vi "Lidar 관심범위 내 데이터(속도결정에 사용).vi"(3 "filter angle(plus)":dbl, 5 "Lidar 오브젝트화 후 배열":dbl[][](array[numeric])) -> (0 "theta":dbl[](array[numeric]), 1 "r":dbl[](array[numeric]), 2 "차량 진행 영역의 장애물":dbl[][](array[numeric]))   [LabVIEW 2016]
uses:
  <vilib>/imath/engines/lvmath2/RunTimeEngine/Managers/WorkSpace/UID Generator.vi
  <vilib>/imath/engines/lvmath2/RunTimeEngine/BuiltInFunctions/size/NIMS_I32Row=size(GM).vi
  <instcachedir>/0/NIMS_I32Row=size(GM)_10ACDCB9F1F84A7E9F42C91D87611FB5.lvgen/NIMS_I32Row=size(GM)_10ACDCB9F1F84A7E9F42C91D87611FB5_001.vi
  <vilib>/imath/engines/lvmath2/RunTimeEngine/RunTimeType/NIMS_RunTimeType_From StrictType (excl LVString).vi
  <instcachedir>/0/NIMS_RunTimeType_From StrictType (excl LVString)_BBF44FB49F834B71AF7A14CCEDF8BECD.lvgen/NIMS_RunTimeType_From StrictType (excl LVString)_BBF44FB49F834B71AF7A14CCEDF8BECD_000.vi
  <vilib>/imath/engines/lvmath2/RunTimeEngine/LocalVariableDefStatement/MC_LocalVariableDefStatement_Display.vi
  <vilib>/imath/engines/lvmath2/RunTimeEngine/IndexRead/NIMS M(S,S).vi
  <instcachedir>/0/NIMS M(S,S)_AC51E74150A542F7991B9634C66F3096.lvgen/NIMS M(S,S)_AC51E74150A542F7991B9634C66F3096_002.vi
  <vilib>/imathl/engines/lvmath/Functions/Error Handling/Create Error.vi
  <vilib>/imath/engines/lvmath2/RunTimeEngine/Managers/SymbolTable/Clear UID.vi
  <vilib>/imath/engines/lvmath2/RunTimeEngine/NodeEndStatement/NIMS_NodeEndStatement_Output.vi
  <instcachedir>/0/NIMS_NodeEndStatement_Output_53EC0D466D134D7ABD903AC30B43404B.lvgen/NIMS_NodeEndStatement_Output_53EC0D466D134D7ABD903AC30B43404B_010.vi
  <vilib>/imath/engines/lvmath2/RunTimeEngine/ErrorHandling/NIMS_Finalize Error.vi
  <vilib>/imath/engines/lvmath2/RunTimeEngine/IndexRead/NIMS M($,S).vi
  <instcachedir>/0/NIMS M($,S)_3E5749BBB62E49528D4765A77F1F6D98.lvgen/NIMS M($,S)_3E5749BBB62E49528D4765A77F1F6D98_000.vi
  <instcachedir>/0/NIMS_NodeEndStatement_Output_53EC0D466D134D7ABD903AC30B43404B.lvgen/NIMS_NodeEndStatement_Output_53EC0D466D134D7ABD903AC30B43404B_005.vi
  <vilib>/imath/engines/lvmath2/RunTimeEngine/Managers/SymbolTable/NIMS_WorkSpace.lvlib
panel:
  out "차량 진행 영역의 장애물 개수":i32
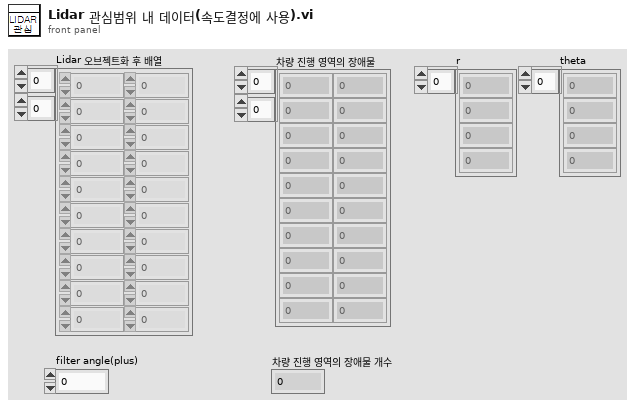
[diagram p1: front panel]
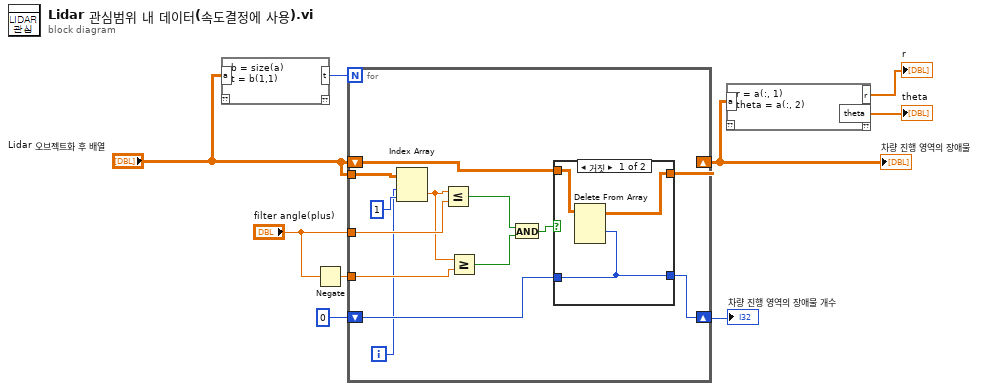
[diagram p0: block diagram]
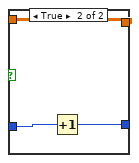
[diagram p2: hidden frame]
diagram:
  n1 = mathscript code="b = size(a)\nt = b(1,1)"("a"="Lidar 오브젝트화 후 배열") -> ("t"=w5:i32)  [unwired: 1 in, 1 out]
  n2 = Negate(x="filter angle(plus)") -> (-x=w8:dbl)
  n3 = for {
    N: w5 -> [_]
    tunnel: "filter angle(plus)" -> [w21]
    tunnel: w8 -> [w19]
    shift-right: [w12] -> w6
    shift-left: 0 ("비활성화된 인덱스 (행)") -> [w14]
    shift-right: [w13] -> w3
    shift-left: "Lidar 오브젝트화 후 배열" -> [w15]
    tunnel: "Lidar 오브젝트화 후 배열" -> [w11]
    i -> [w10]
    n4 = Index Array(array=w11, index (row)=w10, index (col)=1 ("비활성화된 인덱스 (열)")) -> (element=w20:dbl)
    n5 = Less Or Equal?(x=w20, y=w21) -> (x <= y?=w18:bool)
    n6 = Greater Or Equal?(x=w20, y=w19) -> (x >= y?=w17:bool)
    n7 = And(x=w18, y=w17) -> (x .and. y?=w16:bool)
    n8 = case shown="거짓" w16 {
      tunnel: w15 -> [w25 w26]
      tunnel: w14 -> [w23 w28]
      tunnel: [w24 w26] -> w13
      tunnel: [w23 w27] -> w12
      frame False {
        n9 = Delete From Array(array=w25, index (row)=w23) -> (array with subset deleted=w24:dbl[][])  [unwired: 2 in, 1 out]
      }
      frame True {
        n10 = Increment(x=w28) -> (x+1=w27:i32)
      }
    }
  }
  "차량 진행 영역의 장애물" <- w3
  "차량 진행 영역의 장애물 개수" <- w6
  n11 = mathscript code="r = a(:, 1)\ntheta = a(:, 2)"("a"=w3) -> ("r"=→"r":dbl[], "theta"=→"theta":dbl[])  [unwired: 1 in, 1 out]
